vi "unreserve all resources reserved by this node.vi"(8 "error in (no error)":errorcluster, 11 "Item Ref in":T1 format="%.0x") -> (0 "error out":errorcluster, 3 "Item Ref out":T1 format="%.0x")   [LabVIEW 2016, in "FPGA RM System Definition API.lvlib"]
uses:
  FPGA RM System Definition API.lvlib
  <vilib>/NI Veristand/Custom Device API/Custom Device Item Ref.ctl
  <vilib>/NI VeriStand/Custom Device API/Custom Device API.lvlib
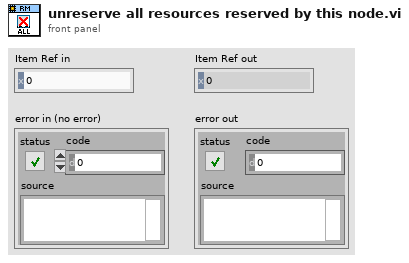
[diagram p1: front panel]
types:
  T1 = typedef "Custom Device API.lvlib/Custom Device Item Ref.ctl" = u64
  T2 = typedef "FPGA RM System Definition API.lvlib/resources.ctl" = cluster{"fpga cd":T1, "resource":T3}
  T3 = typedef "FPGA RM Shared API.lvlib/fpga resource.ctl" = cluster{"name":string, "datatype":string, "channel type":T4, "value":variant, "notes":string}
  T4 = typedef "FPGA RM Shared API.lvlib/Channel Type.ctl" = enum16{"Write Channel", "Read Channel", "Write Waveform", "Read Waveform"}
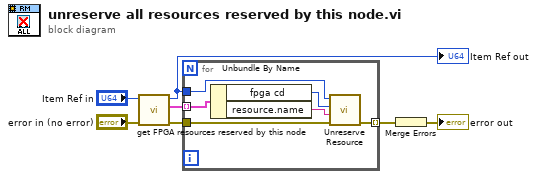
[diagram p0: block diagram]
diagram:
  n1 = call "get FPGA resources reserved by this node.vi"("error in (no error)"="error in (no error)", "Node Ptr"="Item Ref in") -> ("error out"=w1:errorcluster, "reserved resources"=w4:T2[], "Item Ref out"=w5:T1)  [unwired: 7 in]
  "Item Ref out" <- w5
  n2 = for {
    tunnel: w4 -> [w13] mode=indexing
    tunnel: w5 -> [w10]
    tunnel: w1 -> [w9]
    tunnel: [w8] -> w6 mode=indexing
    n3 = Unbundle By Name(w13) -> ("fpga cd"=w11:T1, "resource.name"=w12:string)
    n4 = call "Unreserve Resource.vi"("error in (no error)"=w9, "Name in Bitfile"=w12, "Server Ref in"=w11, "Item Ref in"=w10) -> ("error out"=w8:errorcluster)  [unwired: 6 in, 1 out]
  }
  n5 = Merge Errors(w6) -> (→"error out":errorcluster)
